vi "1 Ball Center Hot.vi"(1 "Run?":bool) -> (0 "Done?":bool)   [LabVIEW 2013]
uses:
  Globals/Homes.vi
  Globals/Useful Values.vi
panel:
  out "Sum":dbl
  out "Ready for Vision?":bool
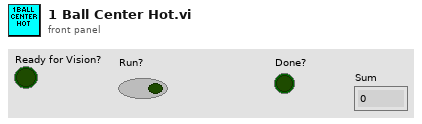
[diagram p1: front panel]
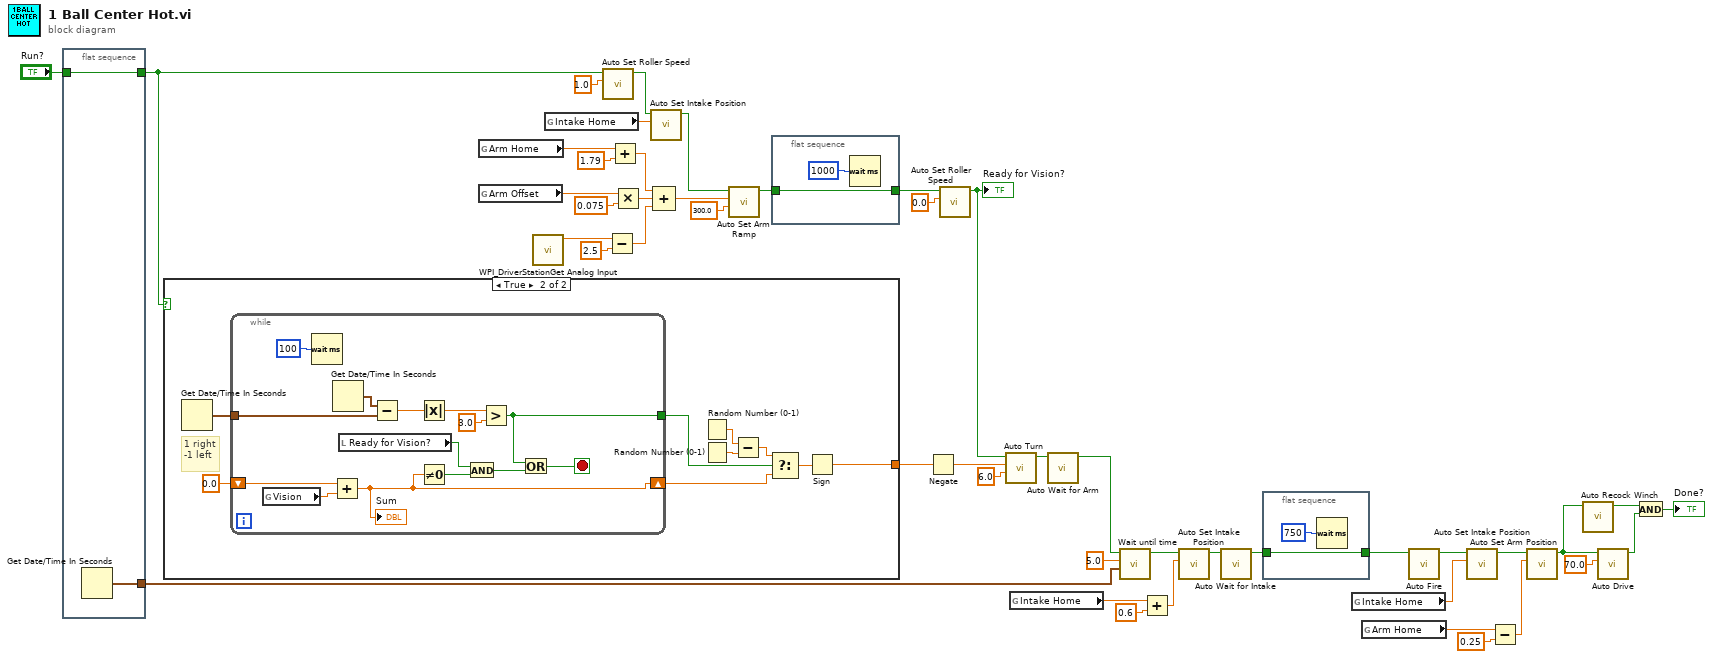
[diagram p0: block diagram]
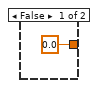
[diagram p2: hidden frame]
diagram:
  n1 = flat-sequence {
    tunnel: "Run?" -> [w48]
    tunnel: [w48] -> w15
    tunnel: [w47] -> w12
    frame #0 {
      n2 = Get Date/Time In Seconds() -> (seconds since 1Jan1904=w47:timestamp)
    }
  }
  n3 = case shown="True" w15 {
    tunnel: [0.0 w50] -> w18
    frame False {
    }
    frame True {
      # "1 right\n-1 left"
      n4 = Get Date/Time In Seconds() -> (seconds since 1Jan1904=w57:timestamp)
      n5 = while {
        shift-right: [w68] -> w52
        shift-left: 0.0 -> [w71]
        tunnel: w57 -> [w66]
        tunnel: [w59] -> w53
        stop <- w61 stop-if-true
        n6 = global read "Useful Values.vi" "Vision"() -> (w72:dbl)
        n7 = Wait (ms)(milliseconds to wait=u32 100) -> ()  [unwired: 1 out]
        n8 = Add(x=w71, y=w72) -> (x+y=w68:dbl)
        "Sum" <- w68
        n9 = Get Date/Time In Seconds() -> (seconds since 1Jan1904=w65:timestamp)
        n10 = local read "Ready for Vision?"() -> (w69:bool)
        n11 = Subtract(x=w65, y=w66) -> (x-y=w64:dbl)
        n12 = Absolute Value(x=w64) -> (abs(x)=w63:dbl)
        n13 = Not Equal To 0?(x=w68) -> (x != 0?=w67:bool)
        n14 = And(x=w69, y=w67) -> (x .and. y?=w60:bool)
        n15 = Greater?(x=w63, y=3.0) -> (0:w59:bool)
        n16 = Or(x=w59, y=w60) -> (x .or. y?=w61:bool)
      }
      n17 = Random Number (0-1)() -> (number: 0 to 1=w54:dbl)
      n18 = Random Number (0-1)() -> (number: 0 to 1=w55:dbl)
      n19 = Subtract(x=w54, y=w55) -> (x-y=w56:dbl)
      n20 = Select(t=w56, s=w53, f=w52) -> (s? t:f=w51:dbl)
      n21 = Sign(1:w51) -> (0:w50:dbl)
    }
  }
  n22 = global read "Homes.vi" "Arm Home"() -> (w9:dbl)
  n23 = global read "Useful Values.vi" "Arm Offset"() -> (w6:dbl)
  n24 = call <vilib>:"WPI_DriverStationGet Analog Input.vi"() -> ("Analog 1 (V)"=w3:dbl)  [unwired: 8 in, 3 out]
  n25 = global read "Homes.vi" "Intake Home"() -> (w40:dbl)
  n26 = call "Auto Set Roller Speed.vi"("Value"=1.0, "Run?"=w15) -> ("Done"=w29:bool)  [unwired: 9 in]
  n27 = Subtract(x=w3, y=2.5) -> (x-y=w2:dbl)
  n28 = Add(x=w9, y=1.79) -> (x+y=w5:dbl)
  n29 = Multiply(x=w6, y=0.075) -> (x*y=w8:dbl)
  n30 = call "Auto Set Intake Position.vi"("Intake Position"=w40, "Run?"=w29) -> ("Done"=w28:bool)  [unwired: 9 in]
  n31 = Compound Arithmetic op=ADD(w5, w8, w2) -> (w1:dbl)
  n32 = call "Auto Set Arm Ramp.vi"("Time (ms)"=300.0, "Arm Position"=w1, "Run?"=w28) -> ("Done"=w20:bool)  [unwired: 8 in]
  n33 = flat-sequence {
    tunnel: w20 -> [w74]
    tunnel: [w74] -> w25
    frame #0 {
      n34 = Wait (ms)(milliseconds to wait=u32 1000) -> ()  [unwired: 1 out]
    }
  }
  n35 = Negate(x=w18) -> (-x=w26:dbl)
  n36 = call "Auto Set Roller Speed.vi"("Value"=0.0, "Run?"=w25) -> ("Done"=w19:bool)  [unwired: 9 in]
  "Ready for Vision?" <- w19
  n37 = call "Auto Turn.vi"("Turn Amount"=6.0, "+/-?"=w26, "Run?"=w19) -> ("Done"=w17:bool)  [unwired: 8 in]
  n38 = global read "Homes.vi" "Intake Home"() -> (w41:dbl)
  n39 = call "Auto Wait for Arm.vi"("Run?"=w17) -> ("Done"=w14:bool)  [unwired: 10 in]
  n40 = call "Wait until time.vi"("Initial Time"=w12, "Time to wait for"=5.0, "Run?"=w14) -> ("Done"=w11:bool)  [unwired: 8 in]
  n41 = Add(x=w41, y=0.6) -> (x+y=w45:dbl)
  n42 = call "Auto Set Intake Position.vi"("Intake Position"=w45, "Run?"=w11) -> ("Done"=w27:bool)  [unwired: 9 in]
  n43 = call "Auto Wait for Intake.vi"("Run?"=w27) -> ("Done"=w34:bool)  [unwired: 10 in]
  n44 = flat-sequence {
    tunnel: w34 -> [w75]
    tunnel: [w75] -> w33
    frame #0 {
      n45 = Wait (ms)(milliseconds to wait=u32 750) -> ()  [unwired: 1 out]
    }
  }
  n46 = global read "Homes.vi" "Intake Home"() -> (w39:dbl)
  n47 = global read "Homes.vi" "Arm Home"() -> (w36:dbl)
  n48 = call "Auto Fire.vi"("Run?"=w33) -> ("Done"=w44:bool)  [unwired: 10 in]
  n49 = call "Auto Set Intake Position.vi"("Intake Position"=w39, "Run?"=w44) -> ("Done"=w43:bool)  [unwired: 9 in]
  n50 = Subtract(x=w36, y=0.25) -> (x-y=w37:dbl)
  n51 = call "Auto Set Arm Position.vi"("Arm Position"=w37, "Run?"=w43) -> ("Done"=w24:bool)  [unwired: 9 in]
  n52 = call "Auto Recock Winch.vi"("Run?"=w24) -> ("Done"=w22:bool)  [unwired: 10 in]
  n53 = call "Auto Drive.vi"("Amount"=70.0, "Run?"=w24) -> ("Done"=w23:bool)  [unwired: 9 in]
  n54 = And(x=w22, y=w23) -> (x .and. y?=→"Done?":bool)
